vi "UnregisterMat_Anything.vi"(6 "AdressOrData":u64 format="%.0x", 8 "error in":errorcluster, 11 "InputDatatype":refnum<class "Anything.lvclass">) -> (0 "error out":errorcluster, 3 "Datatype":refnum<class "Anything.lvclass">)   [LabVIEW 2020, in "OpenLvVision_OpenCv.lvlib"]
doc: "Unregister mat for dll.\nNo malleable to breake vi inlining!"
uses:
  OpenLvVision_OpenCv.lvlib
  Anything.lvclass
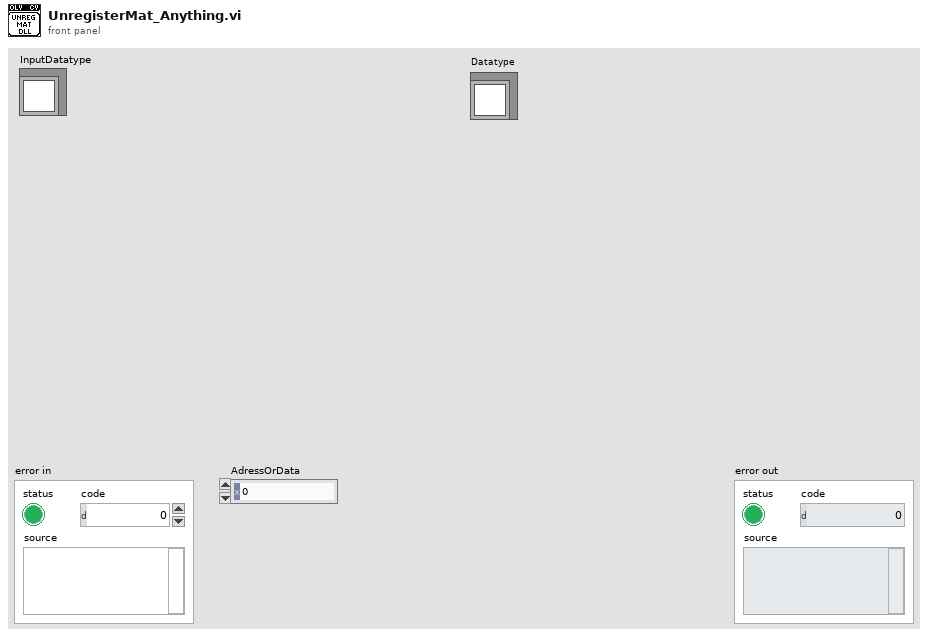
[diagram p1: front panel]
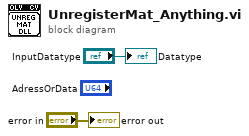
[diagram p0: block diagram]
diagram:
  "Datatype" <- "InputDatatype"
  "error out" <- "error in"
